vi "显示统计.vi"(4 "下棋步数":i32 format="%#_2f", 6 "前面下棋位置":string, 8 "下子方？":i32, 10 "列":i32 format="%#_2f", 11 "行":sgl format="%#_2g") -> (1 "下棋位置":string)   [LabVIEW 2018]
panel:
  out "所下之子":string
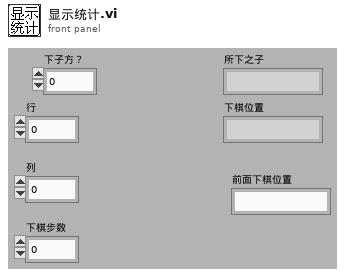
[diagram p1: front panel]
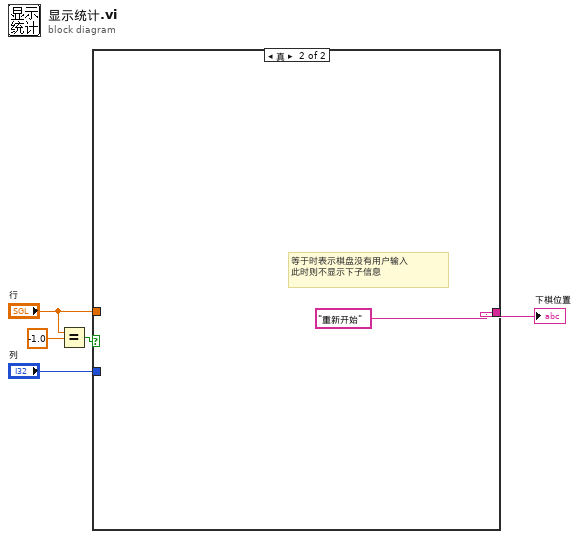
[diagram p0: block diagram]
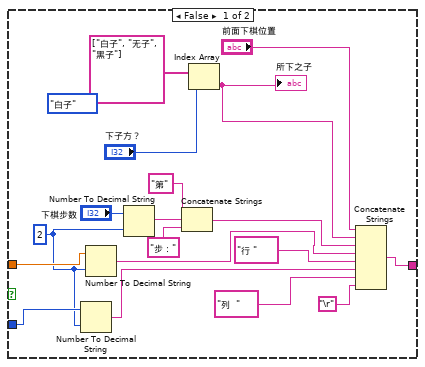
[diagram p2: hidden frame]
diagram:
  n1 = Equal?(x="行", y=sgl -1.0) -> (x = y?=w3:bool)
  n2 = case shown="真" w3 {
    tunnel: "行" -> [w21 _]
    tunnel: "列" -> [w20 _]
    tunnel: [w16 "重新开始"] -> w4
    frame False {
      w10 = i16 2 ("width (-)")
      (unwired) enum16{"白子", "无子", "黑子"}."白子"
      n3 = Number To Decimal String(number=w20, width (-)=w10) -> (decimal integer string=w18:string)
      n4 = Number To Decimal String(number=w21, width (-)=w10) -> (decimal integer string=w19:string)
      n5 = Number To Decimal String(number="下棋步数", width (-)=w10) -> (decimal integer string=w14:string)
      n6 = Concatenate Strings("第" ("string"), w14, "步：" ("string")) -> (w8:string)
      n7 = Index Array(array=string[] ["白子", "无子", "黑子"], index="下子方？") -> (element=w7:string)
      "所下之子" <- w7
      n8 = Concatenate Strings("前面下棋位置", w7, w8, w19, "行 ", w18, "列  ", "\r") -> (w16:string)
    }
    frame True {
      # "等于时表示棋盘没有用户输入\n此时则不显示下子信息"
    }
  }
  "下棋位置" <- w4
